vi "Periodic Tasks.vi"(8 "error in":errorcluster) -> ()   [LabVIEW 2017]
doc: "This VI runs in parallel to other tasks. It can contain as many user-defined periodic loops as you need. These can carry out PID or other sorts of timed response."
uses:
  <vilib>/Rock Robotics/WPI/ThirdParty/Phoenix-LabVIEW/Pigeon IMU/CTRE_PigeonIMU_TareType.ctl
  Robot Global Data.vi
  <vilib>/addons/control/pid/NI_PID_pid.lvlib
  <vilib>/addons/control/pid/pid.llb/PID (DBL).vi
  <vilib>/Rock Robotics/WPI/ThirdParty/Phoenix-LabVIEW/Pigeon IMU/CTRE_PigeonIMU_GetYPR.vi
  <vilib>/Rock Robotics/WPI/Relay/WPI_RelayValue.ctl
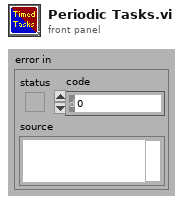
[diagram p1: front panel]
types:
  T1 = typedef "WPI_JoystickDevRef.ctl" = cluster{"Device":T2}
  T2 = typedef "WPI_JoystickDeviceEnum.ctl" = enum16{"USB 0", "USB 1", "USB 2", "USB 3", "USB 4", "USB 5"}
  T3 = typedef "WPI_RobotDriveDevRef.ctl" = cluster{"DevStatus":errorcluster, "Motors[]":T4[], "Square Inputs":bool, "Max Output":dbl}
  T4 = typedef "WPI_MotorControlDeviceRef.ctl" = cluster{"DeviceStatus":errorcluster, "Type":T5, "PWM":cluster{"PWM Channel":T6, "DeadBand":T7}, "CAN":cluster{"Device Number":u8, "SetOutput VI Ref":variant, "GetOutput VI Ref":variant, "Enable VI Ref":variant, "Disable VI Ref":variant, "Data":variant}, "Invert":bool, "DIO PWM":cluster{"PWM \"Enable\" Channel":T6, "DIOChannel":T8, "PWM Rate":dbl}}
  T5 = typedef "WPI_MotorControlType.ctl" = enum16{"PWM", "CAN", "DIO PWM"}
  T6 = typedef "FPGA_DIOPWMChannel.ctl" = enum8{"PWM 0", "PWM 1", "PWM 2", "PWM 3", "PWM 4", "PWM 5", "PWM 6", "PWM 7", "PWM 8", "PWM 9", "PWM MXP 0", "PWM MXP 1", "PWM MXP 2", "PWM MXP 3", "PWM MXP 4", "PWM MXP 5", "PWM MXP 6", "PWM MXP 7", "PWM MXP 8", "PWM MXP 9", "Invalid"}
  T7 = typedef "WPI_PWMDeadband.ctl" = cluster{"Name":string, "maxPositivePwm":i32, "minPositivePwm":i32, "centerPwm":i32, "maxNegativePwm":i32, "minNegativePwm":i32, "angularRange":u16}
  T8 = typedef "FPGA_DIOChannel.ctl" = enum8{"DIO 0", "DIO 1", "DIO 2", "DIO 3", "DIO 4", "DIO 5", "DIO 6", "DIO 7", "DIO 8", "DIO 9", "DIO MXP 0", "DIO MXP 1", "DIO MXP 2", "DIO MXP 3", "DIO MXP 4", "DIO MXP 5", "DIO MXP 6", "DIO MXP 7", "DIO MXP 8", "DIO MXP 9", "DIO MXP 10", "DIO MXP 11", "DIO MXP 12", "DIO MXP 13", "DIO MXP 14", "DIO MXP 15", "SPI Port CS1", "SPI Port CS2", "SPI Port CS3", "SPI Port MISO", "SPI Port MOSI", "Invalid"}
  T9 = cluster{"JoystickDevRef":T1, "RobotDriveDevRef":T3}
  T10 = typedef "CTRE_PigeonIMU_DeviceRef.ctl" = cluster{"DeviceStatus":errorcluster, "Device Number":u8, "Type":T11, "Device ID":u32, "Handle":u64, "UsageFrame":u32, "Library Path":path}
  T11 = typedef "CTRE_PigeonIMU_ConnectionType.ctl" = u32
  T12 = typedef "WPI_RelayValue.ctl" = enum16{"Off", "On", "Forward", "Reverse"}
  T13 = typedef "CTRE_PigeonIMU_TareType.ctl" = u8
  T14 = typedef "WPI_RelayDevRef.ctl" = cluster{"DevStatus":errorcluster, "Relay Channel":T15, "Relay Direction":T16}
  T15 = typedef "FPGA_DIORelayChannel.ctl" = enum8{"Relay 0", "Relay 1", "Relay 2", "Relay 3", "Invalid"}
  T16 = typedef "WPI_RelayDirection.ctl" = enum16{"Both directions", "Forward only", "Reverse only"}
  T17 = enum16{"", "Level 1", "Level 4", "Level 2", "Level 3"}
  T18 = cluster{"proportional gain (Kc)":dbl, "integral time (Ti, min)":dbl, "derivative time (Td, min)":dbl}
  T19 = typedef "WPI_PotentiometerDevRef.ctl" = cluster{"DevStatus":errorcluster, "Analog Channel":T20, "Invert Output":bool}
  T20 = typedef "FPGA_AIChannel.ctl" = enum8{"AI 0", "AI 1", "AI 2", "AI 3", "AI MXP 0", "AI MXP 1", "AI MXP 2", "AI MXP 3", "Invalid"}
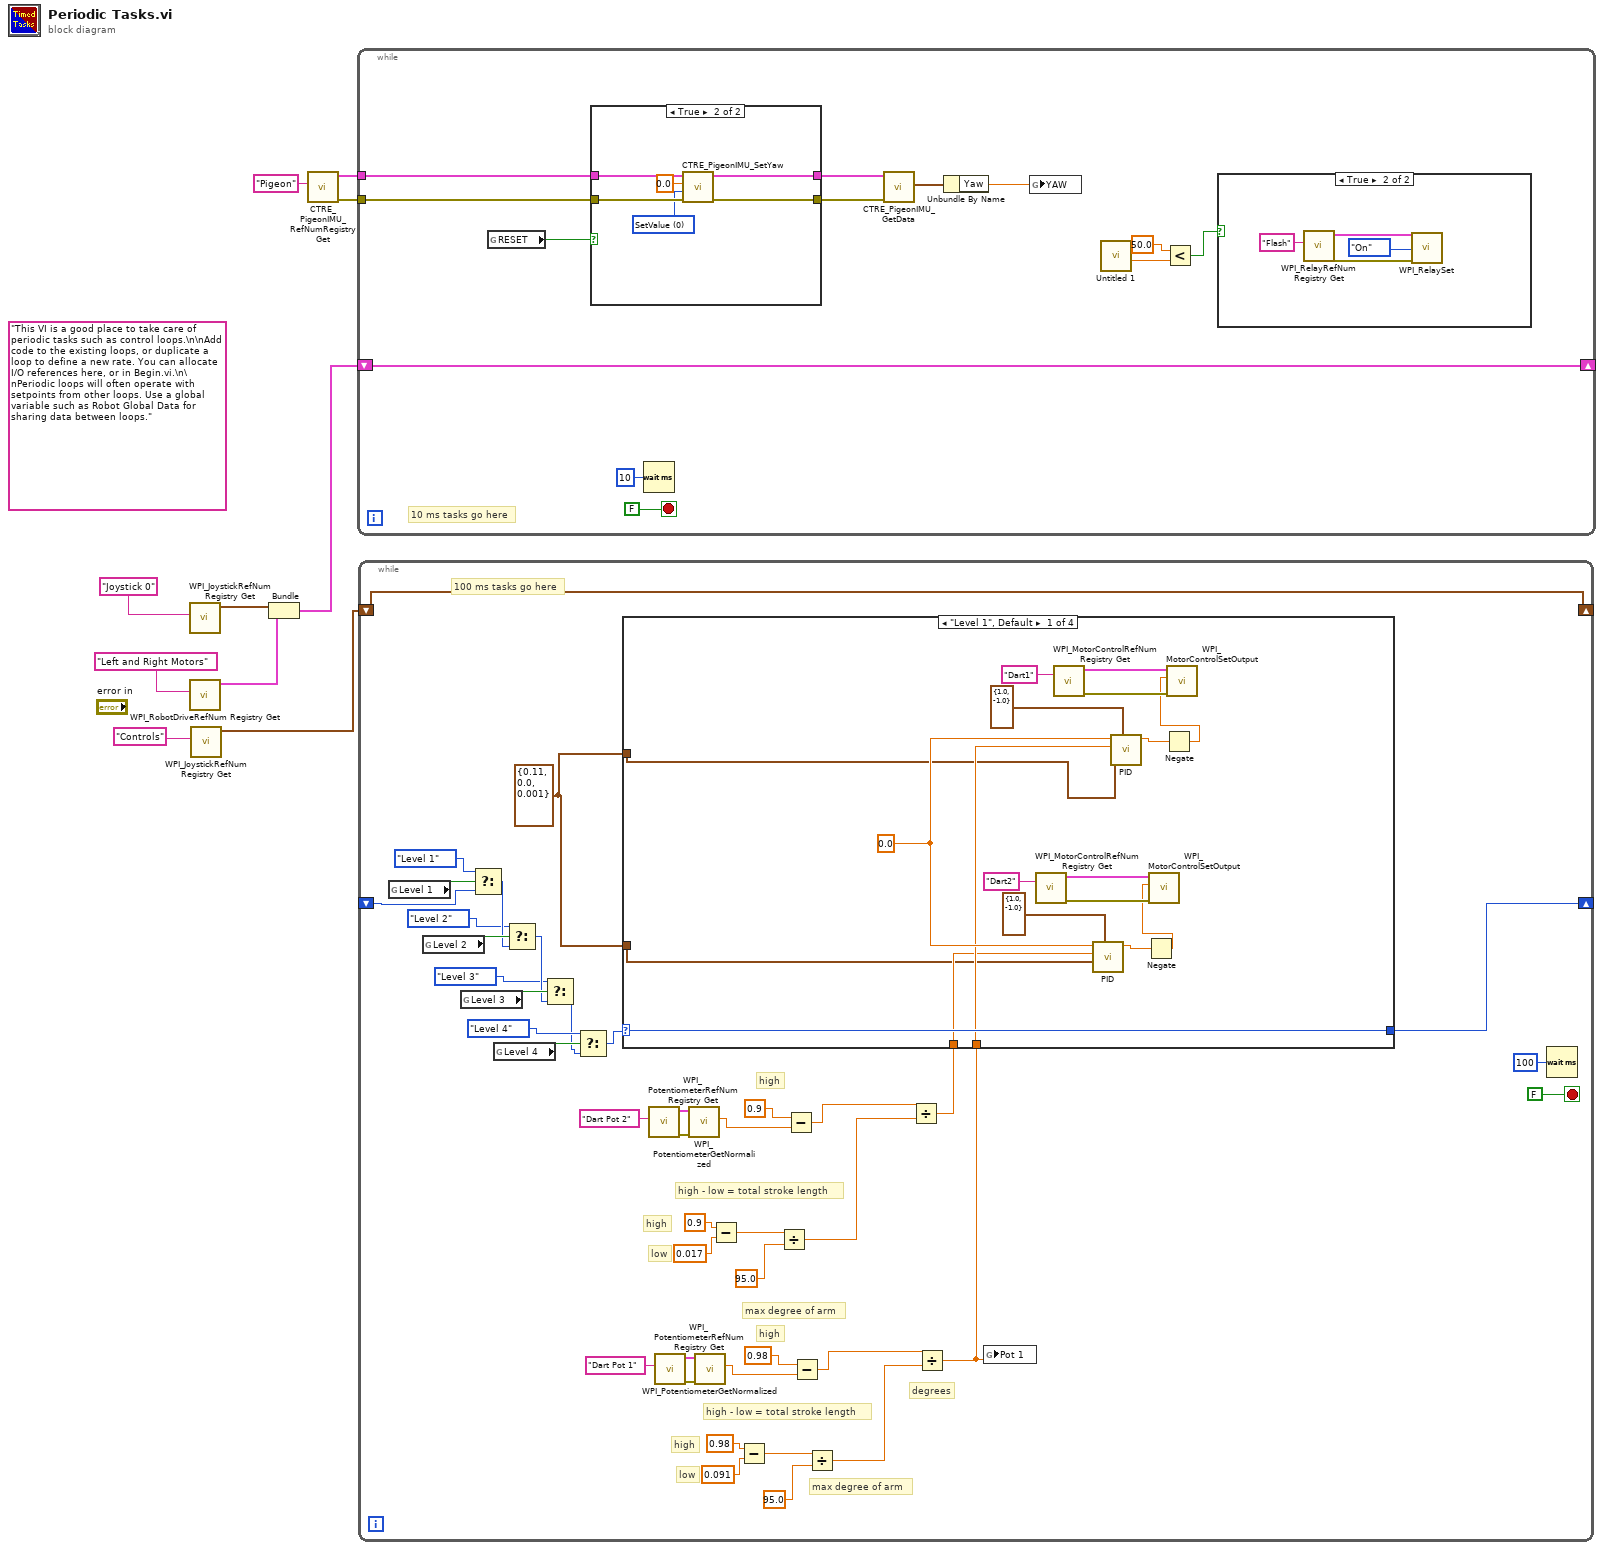
[diagram p0: block diagram]
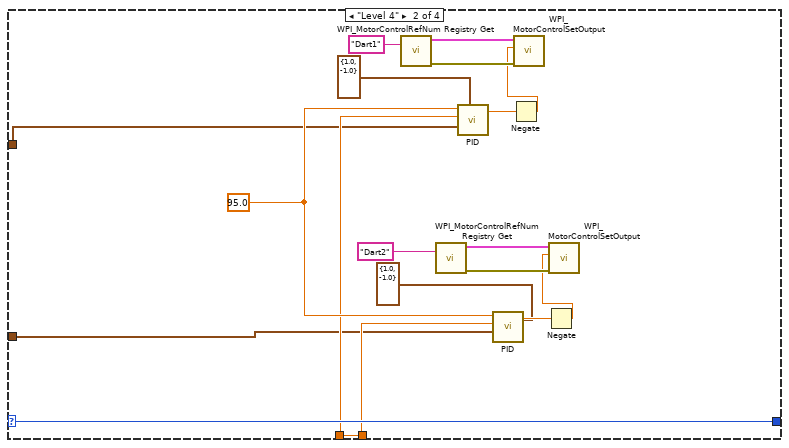
[diagram p2: hidden frame]
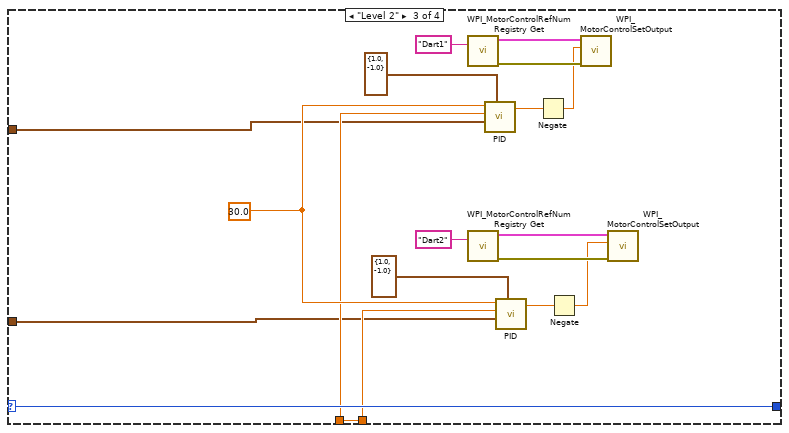
[diagram p3: hidden frame]
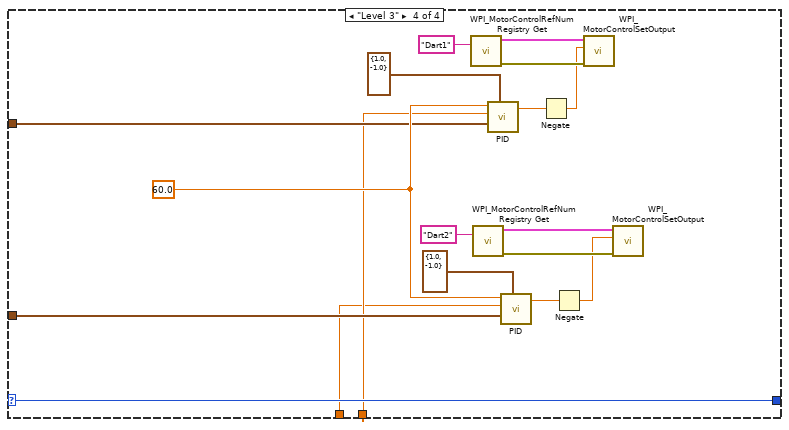
[diagram p4: hidden frame]
diagram:
  (unwired) "This VI is a good place to take care of periodic tasks such as control loops.\n\nAdd code to the existing loops, or duplicate a loop to define a new rate. You can allocate I/O references here, or in Begin.vi.\n\nPeriodic loops will often operate with setpoints from other loops. Use a global variable such as Robot Global Data for sharing data between loops."
  n1 = call <vilib>:"WPI_JoystickRefNum Registry Get.vi"("refnum name"="Joystick 0") -> ("JoystickDevRef"=w8:T1)  [unwired: 1 in, 9 out]
  n2 = call <vilib>:"WPI_RobotDriveRefNum Registry Get.vi"("refnum name"="Left and Right Motors") -> ("RobotDriveDevRef"=w7:T3)  [unwired: 1 in, 9 out]
  n3 = call <vilib>:"WPI_JoystickRefNum Registry Get.vi"("refnum name"="Controls") -> ("JoystickDevRef"=w1:T1)  [unwired: 1 in, 9 out]
  n4 = Bundle("JoystickDevRef"=w8, "RobotDriveDevRef"=w7) -> (w6:T9)  [unwired: 1 out]
  n5 = call <vilib>:"CTRE_PigeonIMU_RefNumRegistryGet.vi"("refnum name"="Pigeon") -> ("error out"=w3:errorcluster, "PigeonIMUDevRef"=w4:T10)  [unwired: 9 in]
  n6 = while {
    shift-right: [w21] -> _
    shift-left: w6 -> [w21]
    tunnel: w4 -> [w20]
    tunnel: w3 -> [w19]
    stop <- FALSE stop-if-true
    # "10 ms tasks go here"
    n7 = global read "Robot Global Data.vi" "RESET"() -> (w18:bool)
    n8 = case shown="True" w18 {
      tunnel: w20 -> [w29 w35]
      tunnel: w19 -> [w28 w34]
      tunnel: [w29 w31] -> w17
      tunnel: [w28 w30] -> w16
      frame False {
      }
      frame True {
        w32 = T13 0 items=["SetValue"=0, "AddOffset"=1, "MatchCompass"=2, "SetOffset"=255] ("TareType (SetValue)")
        n9 = call <vilib>:"CTRE_PigeonIMU_SetYaw.vi"("error in (no error)"=w34, "TareType (SetValue)"=w32, "Value"=0.0, "PigeonIMUDevRef"=w35) -> ("error out"=w30:errorcluster, "PigeonIMUDevRef"=w31:T10)  [unwired: 6 in]
      }
    }
    n10 = Wait (ms)(milliseconds to wait=u32 10) -> ()  [unwired: 1 out]
    n11 = call-poly <vilib>:"CTRE_PigeonIMU_GetData.vi"("error in (no error)"=w16, "PigeonIMUDevRef"=w17) -> ("Yaw Pitch Roll"=w15:cluster{"Yaw":dbl, "Pitch":dbl, "Roll":dbl})  [unwired: 8 in, 1 out]
    n12 = Unbundle By Name(w15) -> ("Yaw"=w14:dbl)
    n13 = global write "Robot Global Data.vi" "YAW"(w14) -> ()
    n14 = call "Untitled 1.vi"() -> ("distance"=w13:dbl)  [unwired: 11 in]
    n15 = Less?(x=50.0, y=w13) -> (x < y?=w11:bool)
    n16 = case shown="True" w11 {
      frame False {
      }
      frame True {
        n17 = call <vilib>:"WPI_RelayRefNum Registry Get.vi"("refnum name"="Flash") -> ("error out"=w24:errorcluster, "RelayDevRef"=w25:T14)  [unwired: 9 in]
        n18 = call <vilib>:"WPI_RelaySet.vi"("error in (no error)"=w24, "RelayValue"=WPI_RelayValue."On", "RelayDevRef"=w25) -> ()  [unwired: 7 in, 2 out]
      }
    }
  }
  n19 = while {
    shift-right: [w75] -> _
    shift-left: w1 -> [w75]
    shift-right: [w73] -> _
    shift-left: _ -> [w45]
    stop <- FALSE stop-if-true
    w43 = T18 {"proportional gain (Kc)"=0.11, "integral time (Ti, min)"=0.0, "derivative time (Td, min)"=0.001} ("PID gains 4")
    # "max degree of arm"
    # "max degree of arm"
    # "low"
    # "high"
    # "high - low = total stroke length"
    # "degrees"
    # "low"
    # "high"
    # "high - low = total stroke length"
    # "high"
    # "high"
    # "100 ms tasks go here"
    n20 = global read "Robot Global Data.vi" "Level 1"() -> (w47:bool)
    n21 = global read "Robot Global Data.vi" "Level 2"() -> (w48:bool)
    n22 = global read "Robot Global Data.vi" "Level 3"() -> (w74:bool)
    n23 = Select(t=T17."Level 1", s=w47, f=w45) -> (s? t:f=w46:T17)
    n24 = global read "Robot Global Data.vi" "Level 4"() -> (w39:bool)
    n25 = Select(t=T17."Level 2", s=w48, f=w46) -> (s? t:f=w44:T17)
    n26 = Select(t=T17."Level 3", s=w74, f=w44) -> (s? t:f=w37:T17)
    n27 = Select(t=T17."Level 4", s=w39, f=w37) -> (s? t:f=w36:T17)
    n28 = call <vilib>:"WPI_PotentiometerRefNum Registry Get.vi"("refnum name"="Dart Pot 2") -> ("error out"=w67:errorcluster, "PotDevRef"=w66:T19)  [unwired: 9 in]
    n29 = call <vilib>:"WPI_PotentiometerRefNum Registry Get.vi"("refnum name"="Dart Pot 1") -> ("error out"=w72:errorcluster, "PotDevRef"=w71:T19)  [unwired: 9 in]
    n30 = call <vilib>:"WPI_PotentiometerGetNormalized.vi"("error in"=w67, "PotDevRef"=w66) -> ("Normalized Value"=w61:dbl)  [unwired: 7 in, 2 out]
    n31 = call <vilib>:"WPI_PotentiometerGetNormalized.vi"("error in"=w72, "PotDevRef"=w71) -> ("Normalized Value"=w62:dbl)  [unwired: 7 in, 2 out]
    n32 = Subtract(x=0.9 ("y"), y=0.017) -> (x-y=w53:dbl)
    n33 = Subtract(x=0.98 ("y"), y=0.091) -> (x-y=w58:dbl)
    n34 = Divide(x=w53, y=95.0) -> (x/y=w51:dbl)
    n35 = Subtract(x=0.9 ("y"), y=w61) -> (x-y=w63:dbl)
    n36 = Subtract(x=0.98 ("y"), y=w62) -> (x-y=w68:dbl)
    n37 = Divide(x=w58, y=95.0) -> (x/y=w56:dbl)
    n38 = Divide(x=w63, y=w51) -> (x/y=w49:dbl)
    n39 = Divide(x=w68, y=w56) -> (x/y=w50:dbl)
    n40 = case shown="\"Level 1\", Default" w36 {
      selector: w36 -> [w95 w100 w131 w135]
      tunnel: [w95 w100 w131 w135] -> w73
      tunnel: w50 -> [w81 w99 w117 w134]
      tunnel: w49 -> [w80 w98 w116 w132]
      tunnel: w43 -> [w79 w96 w114 w137]
      tunnel: w43 -> [w78 w97 w115 w136]
      frame "Level 1", Default {
        w82 = 0.0 ("setpoint")
        n41 = call <vilib>:"WPI_MotorControlRefNum Registry Get.vi"("refnum name"="Dart2") -> ("error out"=w89:errorcluster, "MotorControlDevRef"=w88:T4)  [unwired: 9 in]
        n42 = call <vilib>:"WPI_MotorControlRefNum Registry Get.vi"("refnum name"="Dart1") -> ("error out"=w94:errorcluster, "MotorControlDevRef"=w93:T4)  [unwired: 9 in]
        n43 = call-poly <vilib>:"PID.vi"("output range"=cluster{"output high":dbl, "output low":dbl} {"output high"=1.0, "output low"=-1.0}, "PID gains"=w79, "process variable"=w80, "setpoint"=w82) -> ("output"=w86:dbl)  [unwired: 6 in, 1 out]
        n44 = call-poly <vilib>:"PID.vi"("output range"=cluster{"output high":dbl, "output low":dbl} {"output high"=1.0, "output low"=-1.0}, "PID gains"=w78, "process variable"=w81, "setpoint"=w82) -> ("output"=w91:dbl)  [unwired: 6 in, 1 out]
        n45 = Negate(x=w86) -> (-x=w85:dbl)
        n46 = call <vilib>:"WPI_MotorControlSetOutput.vi"("error in (no error)"=w89, "Output"=w85, "MotorControlDevRef"=w88) -> ()  [unwired: 6 in, 3 out]
        n47 = Negate(x=w91) -> (-x=w90:dbl)
        n48 = call <vilib>:"WPI_MotorControlSetOutput.vi"("error in (no error)"=w94, "Output"=w90, "MotorControlDevRef"=w93) -> ()  [unwired: 6 in, 3 out]
      }
      frame "Level 4" {
        w101 = 95.0 ("setpoint")
        n49 = call <vilib>:"WPI_MotorControlRefNum Registry Get.vi"("refnum name"="Dart1") -> ("error out"=w113:errorcluster, "MotorControlDevRef"=w112:T4)  [unwired: 9 in]
        n50 = call <vilib>:"WPI_MotorControlRefNum Registry Get.vi"("refnum name"="Dart2") -> ("error out"=w108:errorcluster, "MotorControlDevRef"=w107:T4)  [unwired: 9 in]
        n51 = call-poly <vilib>:"PID.vi"("output range"=cluster{"output high":dbl, "output low":dbl} {"output high"=1.0, "output low"=-1.0}, "PID gains"=w97, "process variable"=w99, "setpoint"=w101) -> ("output"=w110:dbl)  [unwired: 6 in, 1 out]
        n52 = call-poly <vilib>:"PID.vi"("output range"=cluster{"output high":dbl, "output low":dbl} {"output high"=1.0, "output low"=-1.0}, "PID gains"=w96, "process variable"=w98, "setpoint"=w101) -> ("output"=w105:dbl)  [unwired: 6 in, 1 out]
        n53 = Negate(x=w110) -> (-x=w109:dbl)
        n54 = call <vilib>:"WPI_MotorControlSetOutput.vi"("error in (no error)"=w113, "Output"=w109, "MotorControlDevRef"=w112) -> ()  [unwired: 6 in, 3 out]
        n55 = Negate(x=w105) -> (-x=w104:dbl)
        n56 = call <vilib>:"WPI_MotorControlSetOutput.vi"("error in (no error)"=w108, "Output"=w104, "MotorControlDevRef"=w107) -> ()  [unwired: 6 in, 3 out]
      }
      frame "Level 2" {
        w118 = 30.0 ("setpoint")
        n57 = call <vilib>:"WPI_MotorControlRefNum Registry Get.vi"("refnum name"="Dart1") -> ("error out"=w130:errorcluster, "MotorControlDevRef"=w129:T4)  [unwired: 9 in]
        n58 = call <vilib>:"WPI_MotorControlRefNum Registry Get.vi"("refnum name"="Dart2") -> ("error out"=w125:errorcluster, "MotorControlDevRef"=w124:T4)  [unwired: 9 in]
        n59 = call-poly <vilib>:"PID.vi"("output range"=cluster{"output high":dbl, "output low":dbl} {"output high"=1.0, "output low"=-1.0}, "PID gains"=w115, "process variable"=w117, "setpoint"=w118) -> ("output"=w127:dbl)  [unwired: 6 in, 1 out]
        n60 = call-poly <vilib>:"PID.vi"("output range"=cluster{"output high":dbl, "output low":dbl} {"output high"=1.0, "output low"=-1.0}, "PID gains"=w114, "process variable"=w116, "setpoint"=w118) -> ("output"=w122:dbl)  [unwired: 6 in, 1 out]
        n61 = Negate(x=w127) -> (-x=w126:dbl)
        n62 = Negate(x=w122) -> (-x=w121:dbl)
        n63 = call <vilib>:"WPI_MotorControlSetOutput.vi"("error in (no error)"=w130, "Output"=w126, "MotorControlDevRef"=w129) -> ()  [unwired: 6 in, 3 out]
        n64 = call <vilib>:"WPI_MotorControlSetOutput.vi"("error in (no error)"=w125, "Output"=w121, "MotorControlDevRef"=w124) -> ()  [unwired: 6 in, 3 out]
      }
      frame "Level 3" {
        w138 = 60.0 ("setpoint")
        n65 = call <vilib>:"WPI_MotorControlRefNum Registry Get.vi"("refnum name"="Dart1") -> ("error out"=w149:errorcluster, "MotorControlDevRef"=w133:T4)  [unwired: 9 in]
        n66 = call <vilib>:"WPI_MotorControlRefNum Registry Get.vi"("refnum name"="Dart2") -> ("error out"=w145:errorcluster, "MotorControlDevRef"=w144:T4)  [unwired: 9 in]
        n67 = call-poly <vilib>:"PID.vi"("output range"=cluster{"output high":dbl, "output low":dbl} {"output high"=1.0, "output low"=-1.0}, "PID gains"=w136, "process variable"=w134, "setpoint"=w138) -> ("output"=w147:dbl)  [unwired: 6 in, 1 out]
        n68 = call-poly <vilib>:"PID.vi"("output range"=cluster{"output high":dbl, "output low":dbl} {"output high"=1.0, "output low"=-1.0}, "PID gains"=w137, "process variable"=w132, "setpoint"=w138) -> ("output"=w142:dbl)  [unwired: 6 in, 1 out]
        n69 = Negate(x=w147) -> (-x=w146:dbl)
        n70 = Negate(x=w142) -> (-x=w141:dbl)
        n71 = call <vilib>:"WPI_MotorControlSetOutput.vi"("error in (no error)"=w149, "Output"=w146, "MotorControlDevRef"=w133) -> ()  [unwired: 6 in, 3 out]
        n72 = call <vilib>:"WPI_MotorControlSetOutput.vi"("error in (no error)"=w145, "Output"=w141, "MotorControlDevRef"=w144) -> ()  [unwired: 6 in, 3 out]
      }
    }
    n73 = global write "Robot Global Data.vi" "Pot 1"(w50) -> ()
    n74 = Wait (ms)(milliseconds to wait=u32 100) -> ()  [unwired: 1 out]
  }
